vi "Query Discr scan step size.vi"(8 "error in (no error)":errorcluster, 10 "i (0)":T1, 11 "VISA resource name":refnum<visa-resource-name>) -> (0 "error out":errorcluster, 2 "output":dbl, 3 "VISA resource name out":refnum<visa-resource-name>)   [LabVIEW 2009, in "SR400.lvlib"]
doc: "DY i { ,v }\nThe DY command sets and reads the discriminator\nscan step size. i = 0,1, or 2 designates\ndiscriminator A,B, or T and is required. If v is\nincluded, the selected discriminator scan step is set\nto v Volts where -0.0200 <= v <= 0.0200. The\nresolution is 0.0002 V (0.2 mV). If v is absent, the\nselected discriminator scan step is returned. The\nscan step may be set and read even if the selected discriminator is in the FIXED mode. Changing the\nscan step during a scan will affect the level for the\nnext count period and all those that follow."
uses:
  SR400.lvlib
  Typedefs.llb/Counter.ctl
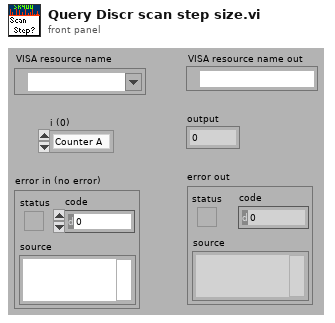
[diagram p1: front panel]
types:
  T1 = typedef "SR400.lvlib/Counter.ctl" = enum16{"Counter A", "Counter B", "Counter T"}
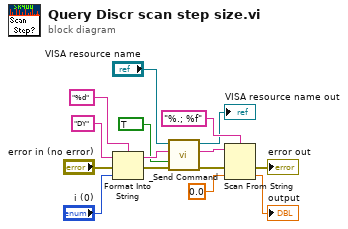
[diagram p0: block diagram]
diagram:
  n1 = Format Into String(format string="%d", initial string="DY" ("command"), error in="error in (no error)", "i (0)") -> (resulting string=w6:string, error out=w5:errorcluster)
  n2 = call "_Send Command.vi"("error in (no error)"=w5, "Query? (F)"=TRUE, "Command"=w6, "VISA resource name"="VISA resource name") -> ("error out"=w2:errorcluster, "Response"=w3:string, "VISA resource name out"=→"VISA resource name out":refnum<visa-resource-name>)  [unwired: 5 out]
  n3 = Scan From String(format string="%.; %f", input string=w3, error in=w2, default 1=0.0 ("default value 1")) -> (error out=→"error out":errorcluster, output 1=→"output":dbl)  [unwired: 1 in, 2 out]
